vi "_RT Read XML Tune Param.vi"(4 "error in":errorcluster, 7 "XML String":string) -> (0 "error out":errorcluster, 2 "TuneParam":T1[](array[typedef]), 3 "Remaining String":string)   [LabVIEW 2015]
uses:
  Type/_RT Active Ch.ctl
  Type/_XML Type.ctl
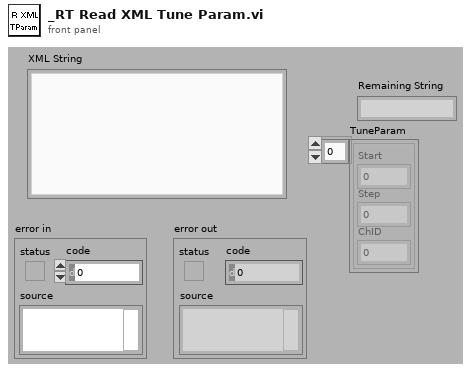
[diagram p1: front panel]
types:
  T1 = typedef "_RT Active Ch.ctl" = cluster{"Start":i32, "Step":i32, "ChID":i32}
  T2 = typedef "_XML Type.ctl" = enum16{"Configuration", "ConTable", "Method", "Experiment", "Mass Range", "Table", "LensTable", "ParamTable", "TuneParam", "MetParam", "MassRange", "LCMethod", "LCMethodFile", "RackType", "Vial", "PlatePos", "InjVol"}
  T3 = typedef "_RT Configuration 2.ctl" = cluster{"Name":string, "Ch#":u8, "Min":dbl, "Max":dbl, "Def+":dbl, "Def-":dbl, "Offset":dbl, "Slope":dbl, "Type":u8, "Description":string, "SettleT":dbl}
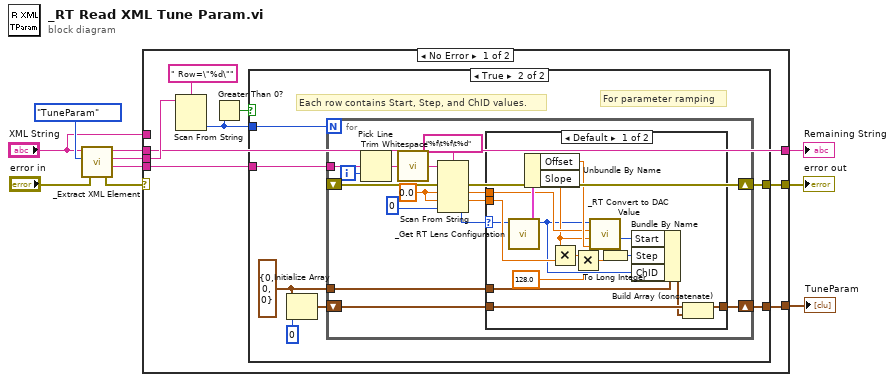
[diagram p0: block diagram]
diagram:
  n1 = call "_Extract XML Element.vi"("error in"="error in", "XML Type"=_XML_Type."TuneParam", "XML String"="XML String") -> ("error out"=w2:errorcluster, "Element"=w8:string, "Attributes"=w7:string, "Remaining String"=w6:string)  [unwired: 1 out]
  n2 = case shown="No Error" w2 {
    selector: w2 -> [_ w58]
    tunnel: [w15 w58] -> w10
    tunnel: w8 -> [w16 _]
    tunnel: w7 -> [w17 _]
    tunnel: w6 -> [w14 _]
    tunnel: "XML String" -> [_ w57]
    tunnel: [w14 w57] -> w4
    tunnel: [w11 _] -> w1
    frame No Error {
      n3 = Scan From String(format string=" Row=\"%d\"", input string=w17) -> (output 1=w12:i32)  [unwired: 2 in, 4 out]
      n4 = Greater Than 0?(x=w12) -> (x > 0?=w13:bool)
      n5 = case shown="True" w13 {
        tunnel: w12 -> [_ w25]
        tunnel: w16 -> [_ w24]
        tunnel: [_ w23] -> w15
        tunnel: [_ w19] -> w11
        frame False {
        }
        frame True {
          w22 = T1 {"Start"=0, "Step"=0, "ChID"=0} ("Active Channel")
          # "For parameter ramping"
          # "Each row contains Start, Step, and ChID values."
          n6 = Initialize Array(w22, 0 ("dimension size")) -> (w20:T1[])
          n7 = for {
            N: w25 -> [_]
            tunnel: w24 -> [w38]
            shift-right: [w35] -> w23
            shift-left: _ -> [w34]
            tunnel: w22 -> [w26]
            shift-right: [w29] -> w19
            shift-left: w20 -> [w30]
            i -> [w37]
            w33 = 0.0 ("Ch#")
            n8 = Pick Line(multi-line string=w38, line index=w37) -> (output string=w39:string)  [unwired: 1 out]
            n9 = call <vilib>:"Trim Whitespace.vi"("string"=w39) -> ("trimmed string"=w36:string)  [unwired: 1 in]
            n10 = Scan From String(format string="%f\t%f\t%d", input string=w36, error in=w34, default 1=w33, default 2=w33, default 3=u8 0 ("Ch#")) -> (error out=w35:errorcluster, output 1=w28:dbl, output 2=w27:dbl, output 3=w31:u8)  [unwired: 1 in, 2 out]
            n11 = case shown="Default" w31 {
              selector: w31 -> [w47 _]
              tunnel: [w45 w56] -> w29
              tunnel: w30 -> [w46 w56]
              tunnel: w28 -> [w53 _]
              tunnel: w27 -> [w52 _]
              tunnel: w26 -> [w50 _]
              frame Default {
                n12 = call "_Get RT Lens Configuration.vi"("Channel #"=w47) -> ("Lens Configuration"=w54:T3)  [unwired: 5 in, 1 out]
                n13 = Unbundle By Name(w54) -> ("Offset"=w55:dbl, "Slope"=w51:dbl)
                n14 = Multiply(x=w51, y=w52) -> (x*y=w43:dbl)
                n15 = Multiply(x=w43, y=128.0) -> (x*y=w41:dbl)
                n16 = call "_RT Convert to DAC Value.vi"("Offset"=w55, "Slop"=w51, "Number"=w53, "Channel"=w47) -> ("DAC Value"=w49:i32)  [unwired: 1 in, 6 out]
                n17 = To Long Integer(number=w41) -> (32bit integer=w48:i32)
                n18 = Bundle By Name(cluster=w50, "Start"=w49, "Step"=w48, "ChID"=w47) -> (w44:T1)
                n19 = Build Array (concatenate)(w46, w44) -> (w45:T1[])
              }
              frame 0..2, 4, 5, 7, 9 {
                # "Cannot ramp\nmass channels"
              }
            }
          }
        }
      }
    }
    frame Error {
    }
  }
  "error out" <- w10
  "Remaining String" <- w4
  "TuneParam" <- w1
